vi "整合数据ID2.vi"(7 "Data in":u8[](array[numeric])) -> (2 "Y":i16, 3 "Y 2":i16, 4 "Y 3":i16, 6 "Y 4":i16, 8 "Y 5":i16, 10 "Y 6":i16, 13 "Y 9":i16, 14 "Y 8":i16, 15 "Y 7":i16)   [LabVIEW 2016]
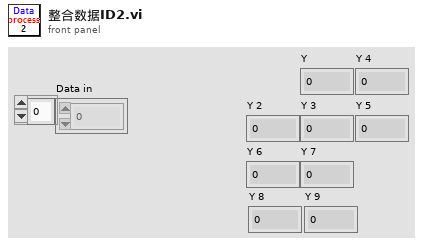
[diagram p1: front panel]
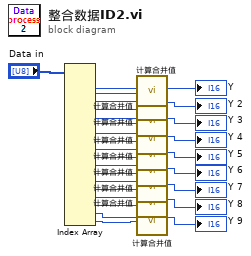
[diagram p0: block diagram]
diagram:
  n1 = Index Array(array="Data in") -> (element #1=w27:u8, element #2=w26:u8, element #3=w25:u8, element #4=w24:u8, element #5=w23:u8, element #6=w22:u8, element #7=w21:u8, element #8=w20:u8, element #9=w19:u8, element #10=w18:u8, element #11=w17:u8, element #12=w16:u8, element #13=w15:u8, element #14=w14:u8, element #15=w13:u8, element #16=w12:u8, element #17=w11:u8, element #18=w10:u8)  [unwired: 18 in]
  n2 = call "计算合并值.vi"("数值H"=w27, "数值L"=w26) -> ("合并数值"=→"Y":i16)  [unwired: 17 in]
  n3 = call "计算合并值.vi"("数值H"=w25, "数值L"=w24) -> ("合并数值"=→"Y 2":i16)  [unwired: 17 in]
  n4 = call "计算合并值.vi"("数值H"=w23, "数值L"=w22) -> ("合并数值"=→"Y 3":i16)  [unwired: 17 in]
  n5 = call "计算合并值.vi"("数值H"=w21, "数值L"=w20) -> ("合并数值"=→"Y 4":i16)  [unwired: 17 in]
  n6 = call "计算合并值.vi"("数值H"=w19, "数值L"=w18) -> ("合并数值"=→"Y 5":i16)  [unwired: 17 in]
  n7 = call "计算合并值.vi"("数值H"=w17, "数值L"=w16) -> ("合并数值"=→"Y 6":i16)  [unwired: 17 in]
  n8 = call "计算合并值.vi"("数值H"=w15, "数值L"=w14) -> ("合并数值"=→"Y 7":i16)  [unwired: 17 in]
  n9 = call "计算合并值.vi"("数值H"=w13, "数值L"=w12) -> ("合并数值"=→"Y 8":i16)  [unwired: 17 in]
  n10 = call "计算合并值.vi"("数值H"=w11, "数值L"=w10) -> ("合并数值"=→"Y 9":i16)  [unwired: 17 in]
